vi "Get PXI8431 Max info.vi"() -> (1 "Slot number":i32[](array[numeric]), 2 "Alias":string[](array[string]))   [LabVIEW 2017]
uses:
  <vilib>/nisyscfg/Close (System).vi
  <vilib>/nisyscfg/nisyscfg.lvlib
  <resource>/objmgr/nisysapi.rc
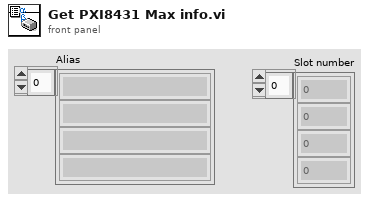
[diagram p1: front panel]
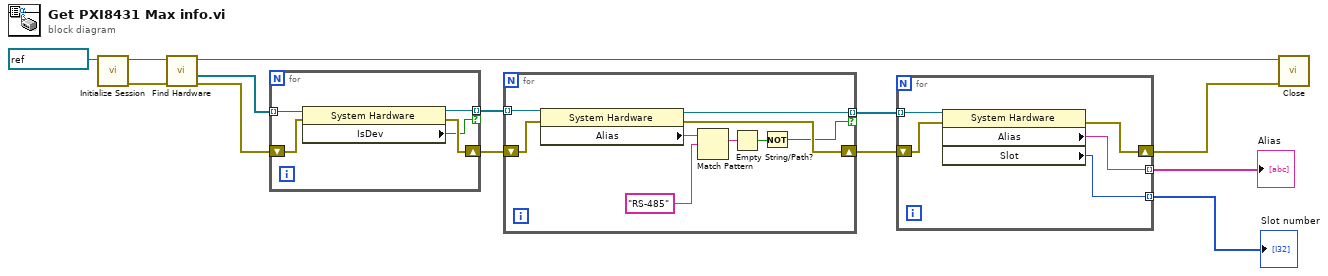
[diagram p0: block diagram]
diagram:
  n1 = call <vilib>:"Initialize Session.vi"("Target (localhost)"=refnum<k21> "localhost") -> ("error out"=w11:errorcluster, "Session out"=w12:refnum<k21>)  [unwired: 9 in]
  n2 = call <vilib>:"Find Hardware.vi"("error in (no error)"=w11, "Session in"=w12) -> ("error out"=w8:errorcluster, "Resources out"=w9:refnum<k20>[], "Session out"=w10:refnum<k21>)  [unwired: 6 in, 1 out]
  n3 = for {
    tunnel: w9 -> [w18] mode=indexing
    shift-right: [w16] -> w6
    shift-left: w8 -> [w17]
    tunnel: [w15] -> w7 mode=indexing if=w14
    n4 = property class="System Hardware"(reference=w18, error in=w17) -> (reference out=w15:refnum<k20>, error out=w16:errorcluster, "IsDev"=w14:bool)
  }
  n5 = for {
    tunnel: w7 -> [w27] mode=indexing
    shift-right: [w21] -> w4
    shift-left: w6 -> [w26]
    tunnel: [w20] -> w5 mode=indexing if=w19
    n6 = property class="System Hardware"(reference=w27, error in=w26) -> (reference out=w20:refnum<k20>, error out=w21:errorcluster, "Alias"=w25:string)
    n7 = Match Pattern(string=w25, regular expression="RS-485") -> (match substring=w23:string)  [unwired: 1 in, 3 out]
    n8 = Empty String/Path?(string/path=w23) -> (empty?=w22:bool)
    n9 = Not(x=w22) -> (.not. x?=w19:bool)
  }
  n10 = for {
    tunnel: w5 -> [w32] mode=indexing
    shift-right: [w29] -> w3
    shift-left: w4 -> [w31]
    tunnel: [w30] -> w2 mode=indexing
    tunnel: [w28] -> w1 mode=indexing
    n11 = property class="System Hardware"(reference=w32, error in=w31) -> (error out=w29:errorcluster, "Alias"=w30:string, "Slot"=w28:i32)  [unwired: 1 out]
  }
  "Alias" <- w2
  "Slot number" <- w1
  n12 = call-poly <vilib>:"Close.vi"("error in (no error)"=w3, "Session in"=w10) -> ()  [unwired: 9 in, 1 out]
